vi "Get Recipe Location Settings.vi"(8 "error in (no error)":errorcluster, 11 "Station Config in":refnum<class "Station Config.lvclass">) -> (0 "error out":errorcluster, 3 "Recipe Locations":T1)   [LabVIEW 2015, in "Station Config.lvlib" / "Station Config.lvclass"]
uses:
  Station Config.lvclass
  Recipe Locations -- Cluster.ctl
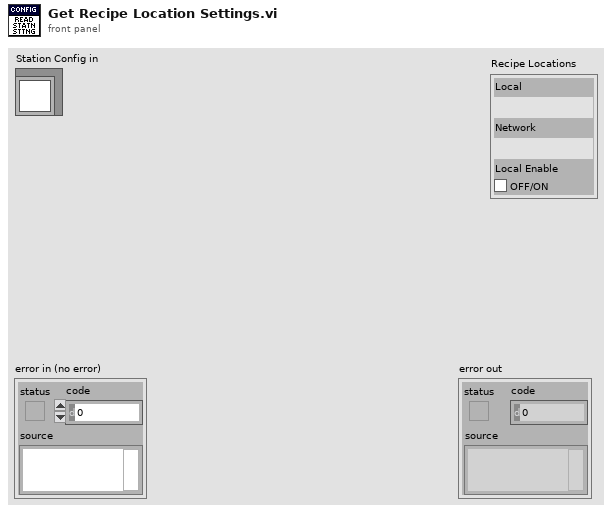
[diagram p1: front panel]
types:
  T1 = typedef "Station Config.lvlib/Station Config.lvclass/Recipe Locations -- Cluster.ctl" = cluster{"Local":path, "Network":path, "Local Enable":bool}
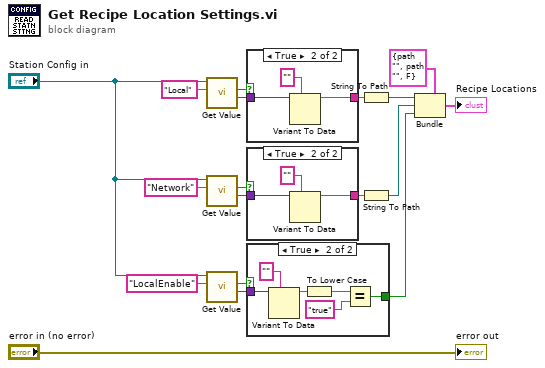
[diagram p0: block diagram]
diagram:
  n1 = call-dynamic "Get Value.vi"("Key"="Local", "Registry in"="Station Config in") -> ("Value"=w16:variant, "found?"=w17:bool)  [unwired: 6 in, 2 out]
  n2 = call-dynamic "Get Value.vi"("Key"="Network", "Registry in"="Station Config in") -> ("Value"=w14:variant, "found?"=w13:bool)  [unwired: 6 in, 2 out]
  n3 = call-dynamic "Get Value.vi"("Key"="LocalEnable", "Registry in"="Station Config in") -> ("Value"=w11:variant, "found?"=w12:bool)  [unwired: 6 in, 2 out]
  n4 = case shown="True" w17 {
    tunnel: w16 -> [_ w21]
    tunnel: [_ w20] -> w8
    frame False {
    }
    frame True {
      n5 = Variant To Data(type="", Variant=w21) -> (data=w20:string)  [unwired: 1 in, 1 out]
    }
  }
  n6 = case shown="True" w13 {
    tunnel: w14 -> [_ w24]
    tunnel: [_ w23] -> w7
    frame False {
    }
    frame True {
      n7 = Variant To Data(type="", Variant=w24) -> (data=w23:string)  [unwired: 1 in, 1 out]
    }
  }
  n8 = case shown="True" w12 {
    tunnel: w11 -> [_ w30]
    tunnel: [_ w25] -> w2
    frame False {
    }
    frame True {
      n9 = Variant To Data(type="", Variant=w30) -> (data=w28:string)  [unwired: 1 in, 1 out]
      n10 = To Lower Case(string=w28) -> (all lower case string=w26:string)
      n11 = Equal?(x=w26, y="true") -> (x = y?=w25:bool)
    }
  }
  n12 = String To Path(string=w8) -> (path=w5:path)
  n13 = String To Path(string=w7) -> (path=w4:path)
  n14 = Bundle(cluster=T1 {"Local"=path "", "Network"=path "", "Local Enable"=FALSE} ("Recipe Locations"), "Local"=w5, "Network"=w4, "Local Enable"=w2) -> (→"Recipe Locations":T1)
  "error out" <- "error in (no error)"
